vi "Shutdown.vi"(8 "error in (no error)":errorcluster, 11 "ATS660 Class in":refnum<class "ATS660 Class.lvclass">) -> (0 "error out":errorcluster, 3 "ATS660 Class out":refnum<class "ATS660 Class.lvclass">)   [LabVIEW 2014, in "ATS660 Class.lvclass"]
uses:
  ATS660 Class.lvclass
  ATS-VI/ATS_ctl/ATS_Async_Ctrl.ctl
  DAQ Class.lvclass
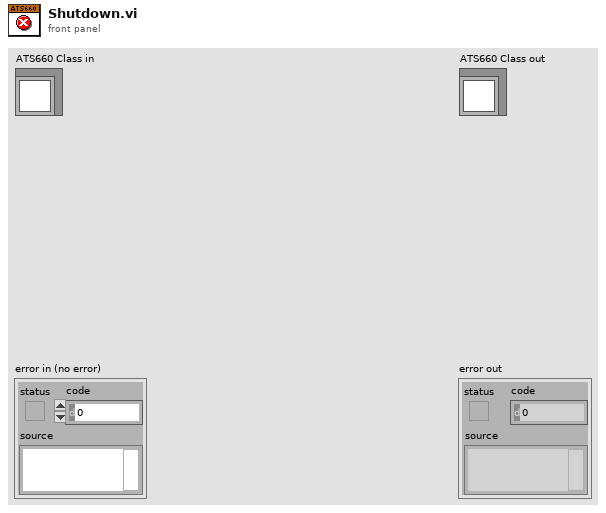
[diagram p1: front panel]
types:
  T1 = typedef "ATS_Async_Ctrl.ctl" = enum16{"SetupDMA", "StartCapture", "Get", "Get_Stream", "Abort", "Stop"}
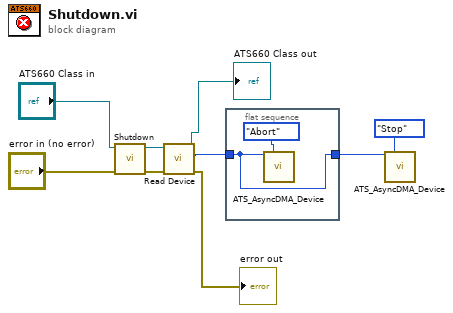
[diagram p0: block diagram]
diagram:
  n1 = call-parent "Shutdown.vi"("error in (no error)"="error in (no error)", "DAQ Class in"="ATS660 Class in") -> ("error out"=w6:errorcluster, "DAQ Class out"=w7:refnum<class "ATS660 Class.lvclass">)  [unwired: 8 in]
  n2 = call-dynamic "Read Device.vi"("error in (no error)"=w6, "ATS660 Class in"=w7) -> ("error out"=→"error out":errorcluster, "Device"=w5:i32, "ATS660 Class out"=→"ATS660 Class out":refnum<class "ATS660 Class.lvclass">)  [unwired: 7 in]
  n3 = flat-sequence {
    tunnel: w5 -> [w10]
    tunnel: [w10] -> w4
    frame #0 {
      n4 = call "ATS_AsyncDMA_Device.vi"("DeviceIn"=w10, "ATS_Async_Ctrl"=ATS_Async_Ctrl."Abort") -> ()  [unwired: 9 in, 5 out]
    }
  }
  n5 = call "ATS_AsyncDMA_Device.vi"("DeviceIn"=w4, "ATS_Async_Ctrl"=ATS_Async_Ctrl."Stop") -> ()  [unwired: 9 in, 5 out]
